vi "AMI1700_get.vi"(8 "error in":errorcluster, 10 "string in":string, 11 "VISA in":refnum<visa-resource-name>) -> (0 "error out":errorcluster, 2 "string out":string, 3 "VISA out":refnum<visa-resource-name>)   [LabVIEW 2019]
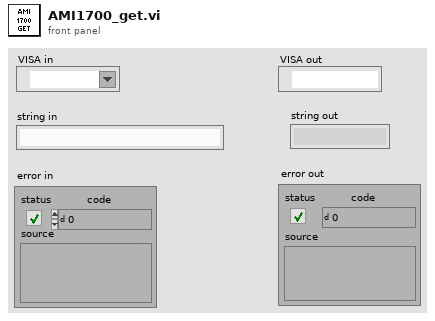
[diagram p1: front panel]
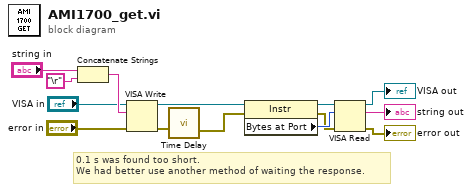
[diagram p0: block diagram]
diagram:
  # "0.1 s was found too short.\nWe had better use another method of waiting the response."
  n1 = Concatenate Strings("string in", "\r") -> (w10:string)
  n2 = VISA Write(VISA resource name="VISA in", write buffer=w10, error in (no error)="error in") -> (VISA resource name out=w14:refnum<visa-resource-name>, error out=w6:errorcluster)  [unwired: 1 out]
  n3 = call "Time Delay"("error in (no error)"=w6) -> ("error out"=w5:errorcluster)  [unwired: 10 in]
  n4 = property class="Instr"(reference=w14, error in=w5) -> (reference out=w13:refnum<visa-resource-name>, error out=w7:errorcluster, "Bytes at Port"=w9:u32)
  n5 = VISA Read(VISA resource name=w13, byte count=w9, error in (no error)=w7) -> (VISA resource name out=→"VISA out":refnum<visa-resource-name>, read buffer=→"string out":string, error out=→"error out":errorcluster)  [unwired: 1 out]
